vi "test-timer-2-DUP_DELETE.vi"() -> ()   [LabVIEW 2019]
uses:
  <vilib>/Rock Robotics/WPI/ThirdParty/JAS_Junk/TrajLib/Trajectory_Library.lvlib
panel:
  out "T0 - Diff = 5.0":dbl
  # "Timer test -- Note this doesn't really test the Timer functionality, \nonly the get time functionality."
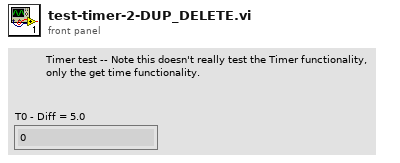
[diagram p1: front panel]
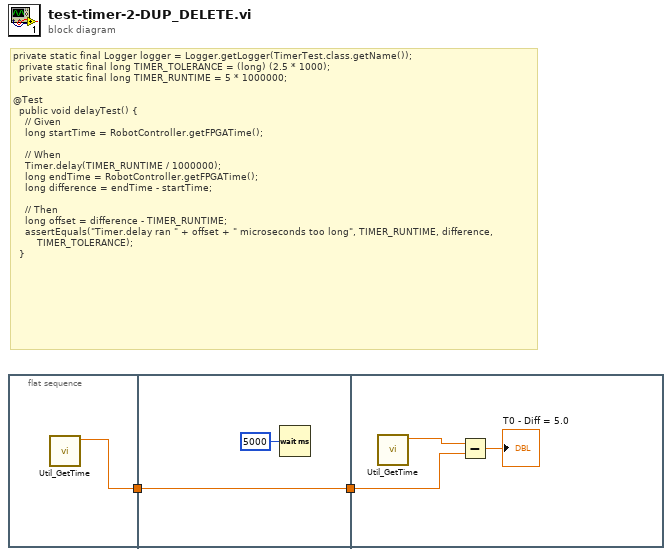
[diagram p0: block diagram]
diagram:
  # "private static final Logger logger = Logger.getLogger(TimerTest.class.getName());\n  private static final long TIMER_TOLERANCE = (long) (2.5 * 1000);\n  private static final long TIMER_RUNTIME = 5 * 1000000;\n\n@Test\n  public void delayTest() {\n    // Given\n    long startTime = RobotController.getFPGATime();\n\n    // When\n    Timer.delay(TIMER_RUNTIME / 1000000);\n    long endTime = RobotController.getFPGATime();\n    long difference = endTime - startTime;\n\n    // Then\n    long offset = difference - TIMER_RUNTIME;\n    assertEquals(\"Timer.delay ran \" + offset + \" microseconds too long\", TIMER_RUNTIME, difference,\n        TIMER_TOLERANCE);\n  }"
  n1 = flat-sequence {
    tunnel: [w3] -> w1
    tunnel: [w4] -> w2
    tunnel: w1 -> [w4]
    tunnel: w2 -> [w7]
    frame #0 {
      n2 = call <vilib>:"Util_GetTime.vi"() -> ("FPGA_Time_Seconds"=w3:dbl)  [unwired: 10 in, 1 out]
    }
    frame #1 {
      n3 = Wait (ms)(milliseconds to wait=u32 5000) -> ()  [unwired: 1 out]
    }
    frame #2 {
      n4 = call <vilib>:"Util_GetTime.vi"() -> ("FPGA_Time_Seconds"=w8:dbl)  [unwired: 10 in, 1 out]
      n5 = Subtract(x=w8, y=w7) -> (x-y=→"T0 - Diff = 5.0":dbl)
    }
  }
